vi "1.vi"() -> ()   [LabVIEW 2017]
panel:
  out "数值":dbl
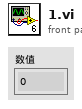
[diagram p1: front panel]
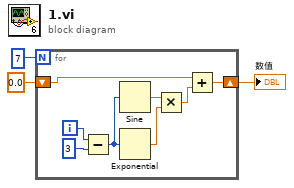
[diagram p0: block diagram]
diagram:
  n1 = for {
    N: 7 -> [_]
    shift-right: [w4] -> w1
    shift-left: 0.0 -> [w5]
    i -> [w11]
    n2 = Subtract(x=w11, y=3) -> (x-y=w9:i32)
    n3 = Sine(x=w9) -> (sin(x)=w8:dbl)
    n4 = Exponential(1:w9) -> (0:w7:dbl)
    n5 = Multiply(x=w8, y=w7) -> (x*y=w6:dbl)
    n6 = Add(x=w5, y=w6) -> (x+y=w4:dbl)
  }
  "数值" <- w1
